vi "Is Scalar Vector Matrix.vi"(11 "octave sizes":i32[](array[numeric])) -> (0 "is >2d matrix?":bool, 1 "is matrix?":bool, 2 "is vector?":bool, 3 "is scalar?":bool, 4 "row vector?":bool, 5 "vector length":i32=-1)   [LabVIEW 2020, in "GOLPI library.lvlib"]
doc: "Returns if object determined by sizes specified on input is scalar, vector or matrix. If vector, returns if is row vector and returns length of the vector. Sizes are in GNU Octave metrics (no elements with zero indexes). Mathematically, x=[1] is scalar and also is vector and also is matrix, however this vi returns only one possibility."
uses:
  GOLPI library.lvlib
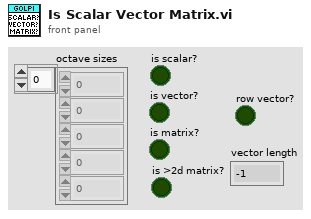
[diagram p1: front panel]
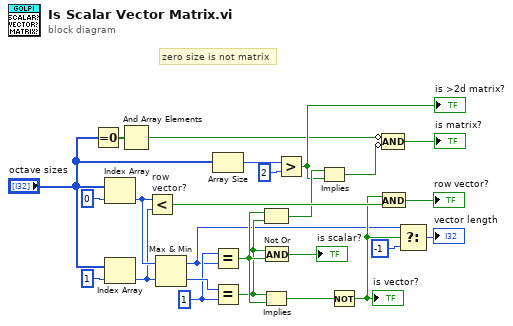
[diagram p0: block diagram]
diagram:
  w20 = 1 ("y")
  # "zero size is not matrix"
  n1 = Equal To 0?(x="octave sizes") -> (x = 0?=w4:bool[])
  n2 = Index Array(array="octave sizes", index=0) -> (element=w23:i32)
  n3 = Index Array(array="octave sizes", index=1) -> (element=w22:i32)
  n4 = And Array Elements(Boolean array=w4) -> (logical AND=w3:bool)
  n5 = Less? "row\nvector?"(x=w23, y=w22) -> (x < y?=w13:bool)
  n6 = Max & Min(x=w23, y=w22) -> (max(x,y)=w8:i32, min(x,y)=w21:i32)
  n7 = Array Size(array="octave sizes") -> (size(s)=w14:i32)
  n8 = Equal?(x=w20, y=w8) -> (x = y?=w17:bool)
  n9 = Equal?(x=w21, y=w20) -> (x = y?=w15:bool)
  n10 = Not Or(1:w15, 2:w17) -> (0:w11:bool)
  n11 = Implies(1:w17, 2:w15) -> (0:w16:bool)
  n12 = And(x=w15, y=w17) -> (x .and. y?=→"is scalar?":bool)
  n13 = Greater?(x=w14, y=2) -> (0:w10:bool)
  "is >2d matrix?" <- w10
  n14 = Implies(1:w10, 2:w11) -> (0:w1:bool)
  n15 = Not(x=w16) -> (.not. x?=w9:bool)
  "is vector?" <- w9
  n16 = And(x=w9, y=w13) -> (x .and. y?=→"row vector?":bool)
  n17 = Compound Arithmetic op=AND(invert w3, invert w1) -> (→"is matrix?":bool)
  n18 = Select(t=w8, s=w9, f=-1) -> (s? t:f=→"vector length":i32)
